vi "asdf2.vi"() -> ()   [LabVIEW 2018]
uses:
  Main/Setting.ctl
  Main/Main.lvlib
  53e0e78a-dd2b-405a-b6bc-bac7bb84a88a.vi
  Cfg/Operation.ctl
  Cfg/Cfg.lvlib
panel:
  in  "Tree":string(tree)
  out "Picture":picture
  in  "Enum":enum16{"Hello", "World", "Item 2", "Item 3"}(ring)
  in  "Numeric":i32
  in  "Title":string
  in  "Hide Top Level VI":bool
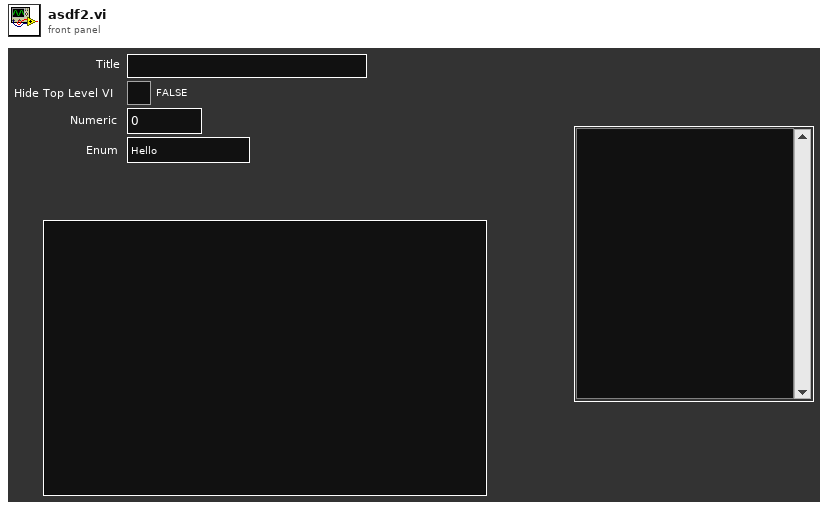
[diagram p1: front panel]
types:
  T1 = typedef "Cfg.lvlib/Operation.ctl" = enum8{"Read or Create", "Read", "Write"}
  T2 = typedef "Main.lvlib/Setting.ctl" = enum8{"noop", "application/title", "application/hide_top_vi", "application/numeric", "application/enum"}
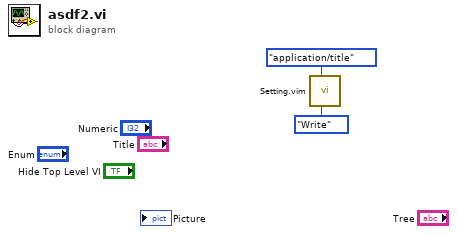
[diagram p0: block diagram]
diagram:
  n1 = call "Setting.vim"("Operation (Read or Create)"=Operation."Write", "Key"=Setting."application/title") -> ()  [unwired: 7 in, 3 out]
